vi "Apply Prefs.vi"(8 "error in (no error)":errorcluster, 11 "GUI Helper in":refnum<class "MessageQ.lvclass">) -> (0 "error out":errorcluster, 3 "GUI Helper out":refnum<class "MessageQ.lvclass">)   [LabVIEW 2020, in "VolatusGUI.lvlib" / "GUI Helper.lvclass"]
uses:
  GUI Helper.lvclass
  Volatus/MessageQ/MessageQ.lvclass
  Volatus/MessageQ/MessageQ.lvclass/MessageQ.ctl
  GUI Helper.lvclass/GUI Helper.ctl
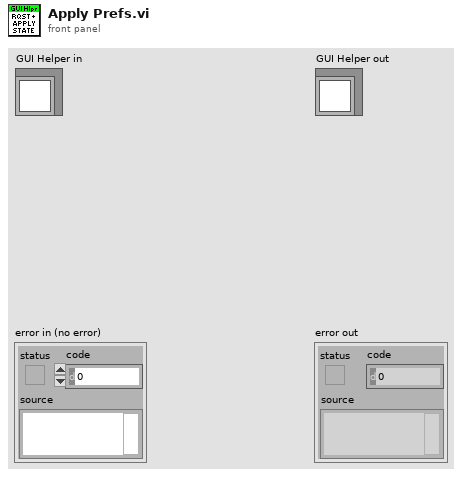
[diagram p1: front panel]
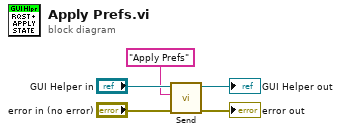
[diagram p0: block diagram]
diagram:
  n1 = call "Send.vi"("error in (no error)"="error in (no error)", "ID"="Apply Prefs", "MessageQ in"="GUI Helper in") -> ("error out"=→"error out":errorcluster, "MessageQ out"=→"GUI Helper out":refnum<class "MessageQ.lvclass">)  [unwired: 7 in]
